vi "HEWH RLT Calculate Start Stop Draw Counts.vi"(8 "Error In":errorcluster, 11 "Test Sequence In":T1[](array[typedef]) {"Time" format="%<%H:%M:%S>t"}) -> (0 "Error Out":errorcluster, 1 "Finish Draw Count":i32[](array[numeric]), 2 "Start Draw Count":i32[](array[numeric]), 3 "Test Sequence Out":T1[](array[typedef]) {"Time" format="%<%H:%M:%S>t"})   [LabVIEW 2019]
uses:
  Type Definitions/PRAT Test.ctl
  Utility/Save File/File Setup (Public)/Type Definition/Save File HEWH Heating Control Mode.ctl
  Draw Water Specific/Type Definitions/Terminate Draw Conditions.ctl
  Type Definitions/HEWH Start Conditions.ctl
  Draw Water Specific/Type Definitions/Check Special Condtions.ctl
  Draw Water Specific/Type Definitions/HEWH Special Condition Check.ctl
  Type Definitions/HEWH Draw Flag ENUM.ctl
  Utility/Save File/File Setup.lvlib
panel:
  out "Total Cycles":i32
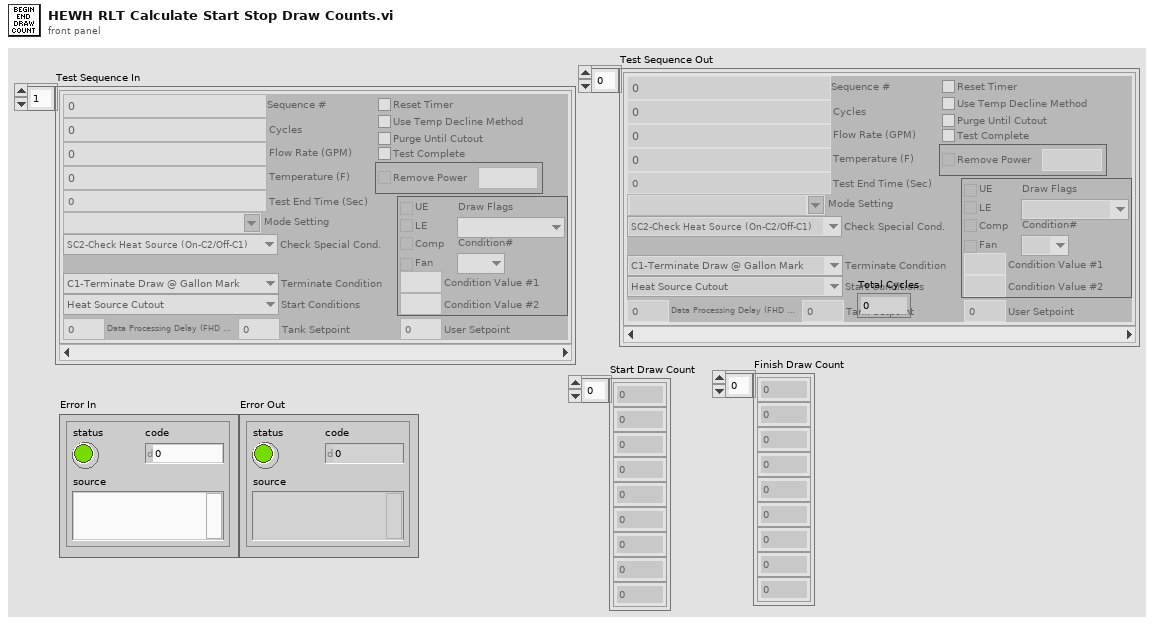
[diagram p1: front panel]
types:
  T1 = typedef "PRAT Test.ctl" = cluster{"Sequence #":dbl, "Cycles":i32, "Mode Setting":T2, "Flow Rate (GPM)":dbl, "Temperature (F)":dbl, "Reset Timer":bool, "Use Temp Decline Method":bool, "Terminate Condition":T3, "Condition Value #1":dbl, "UE":bool, "LE":bool, "Comp":bool, "Fan":bool, "Test End Time (Sec)":dbl, "Purge Until Cutout":bool, "Start Conditions":T4, "Condition Value #2":dbl, "Remove Power":bool, "Time":dbl, "Check Special Cond.":T5, "Condition#":T6, "Draw Flags":T7, "Data Processing Delay (FHD 15sec, UEF 5 Sec)":dbl, "Test Complete":bool, "User Setpoint":dbl, "Tank Setpoint":dbl}
  T2 = typedef "File Setup.lvlib/Save File HEWH Heating Control Mode.ctl" = string
  T3 = typedef "Terminate Draw Conditions.ctl" = enum16{"C1-Terminate Draw @ Gallon Mark", "C2-Special Last Draw (HU Test)", "C3-RTD Out <=", "C4-Mean Tank Temp <=", "C5-Decrease RTD Out (Deg F)", "C6-Time (Seconds)", "C7-Until Any Heat Source", "C8-Specific Heat Source", "C9-Do Nothing", "C10-Inlet Outlet RTD Temp Delta"}
  T4 = typedef "HEWH Start Conditions.ctl" = enum16{"Heat Source Cutout", "At Time (Seconds)", "Every X (Seconds)", "T2 >= X° Below Setpoint", "Seconds From Complete", "Wait for LE & Comp Cutout", "Wait for Comp Cutout", "Wait for LE Cutout", "Wait for UE Cutout", "Start Immediately"}
  T5 = typedef "Check Special Condtions.ctl" = enum16{"SC1-Do Nothing", "SC2-Check Heat Source (On-C2/Off-C1)", "SC3-Check Skip Condition", "SC4-Check Heat Source ON/Fail", "SC5-Keep Draw Valves Open", "SC6-Skip Purge"}
  T6 = typedef "HEWH Special Condition Check.ctl" = enum16{"N/A", "C1", "C2", "Reset/Fail", "Skip Draw Sequence"}
  T7 = typedef "HEWH Draw Flag ENUM.ctl" = enum16{"N/A", "None(0)", "Sml(1)", "Med(2)", "SmlMed(3)", "Lrg(4)", "SmlLrg(5)", "MedLrg(6)", "SmlMedLrg(7)"}
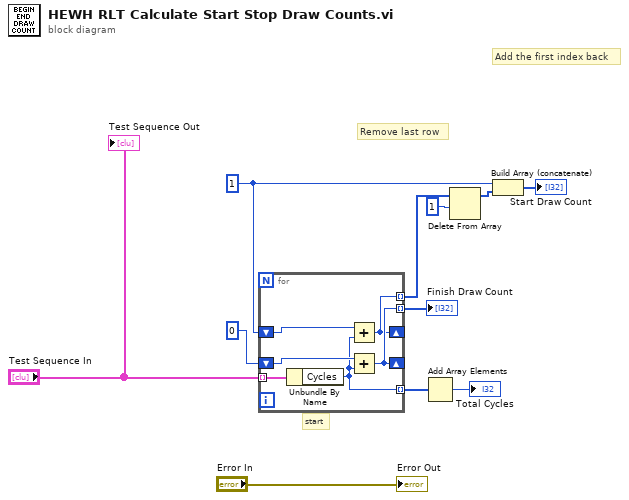
[diagram p0: block diagram]
diagram:
  w8 = 1
  # "Add the first index back"
  # "Remove last row"
  # "start"
  n1 = for {
    tunnel: "Test Sequence In" -> [w17] mode=indexing
    shift-right: [w15] -> _
    shift-left: 0 -> [w16]
    tunnel: [w15] -> w9 mode=indexing
    shift-right: [w13] -> _
    shift-left: w8 -> [w14]
    tunnel: [w13] -> w5 mode=indexing
    tunnel: [w12] -> w2 mode=indexing
    n2 = Unbundle By Name(w17) -> ("Cycles"=w12:i32)
    n3 = Add(x=w14, y=w12) -> (x+y=w13:i32)
    n4 = Add(x=w16, y=w12) -> (x+y=w15:i32)
  }
  "Finish Draw Count" <- w9
  n5 = Add Array Elements(numeric array=w2) -> (sum=→"Total Cycles":i32)
  n6 = Delete From Array(array=w5, length=1) -> (array with subset deleted=w7:i32[])  [unwired: 1 in, 1 out]
  n7 = Build Array (concatenate)(w8, w7) -> (→"Start Draw Count":i32[])
  "Error Out" <- "Error In"
  "Test Sequence Out" <- "Test Sequence In"
